vi "HFRR ADV v05 new software.vi"() -> ()   [LabVIEW 2025] (continued)
                n290 = local write "Command"(w384) -> ()
              }
              frame #2 {
                n291 = Wait (ms)(milliseconds to wait=u32 1500) -> ()  [unwired: 1 out]
              }
              frame #3 {
                n292 = local write "Command"("HE;1" ("Command")) -> ()
              }
              frame #4 {
                n293 = Wait (ms)(milliseconds to wait=u32 1500) -> ()  [unwired: 1 out]
              }
            }
          }
          frame False {
            n294 = stacked-sequence {
              frame #0 {
                n295 = Wait (ms)(milliseconds to wait=u32 1500) -> ()  [unwired: 1 out]
              }
              frame #1 {
                n296 = Concatenate Strings("ST;" ("Command"), "0" ("string")) -> (w393:string)
                n297 = local write "Command"(w393) -> ()
              }
              frame #2 {
                n298 = Wait (ms)(milliseconds to wait=u32 1500) -> ()  [unwired: 1 out]
              }
              frame #3 {
                n299 = local write "Command"("HE;0" ("Command")) -> ()
              }
              frame #4 {
                n300 = Wait (ms)(milliseconds to wait=u32 1500) -> ()  [unwired: 1 out]
              }
            }
          }
        }
      }
      event "Headen Service Button": Value Change {
        n301 = event-data() -> ()  [unwired: 1 in, 6 out]
        n302 = local read "Headen Service Button"() -> (w398:bool)
        n303 = case shown="True" w398 {
          frame False {
            n304 = property on="Password 3" class="Clust (strict)"("Visible"=FALSE) -> ()  [unwired: 2 in, 2 out]
            n305 = property on="Service Password Log" class="Str"("Visible"=FALSE) -> ()  [unwired: 2 in, 2 out]
          }
          frame True {
            n306 = property on="Password 3" class="Clust (strict)"("Visible"=TRUE) -> ()  [unwired: 2 in, 2 out]
            n307 = property on="Service Password Log" class="Str"("Visible"=TRUE) -> ()  [unwired: 2 in, 2 out]
          }
        }
      }
      event "Password 3.Service Password": Value Change {
        n308 = event-data() -> ()  [unwired: 1 in, 6 out]
        n309 = Unbundle By Name("Password 3") -> ("Service Password"=w405:string)
        n310 = call <vilib>:"Trim Whitespace.vi"("string"=w405) -> ("trimmed string"=w403:string)  [unwired: 1 in]
        n311 = Equal?(x=w403, y="Service@123") -> (x = y?=w404:bool)
        n312 = case shown="False" w404 {
          selector: w404 -> [w409 w411]
          frame False {
            n313 = local write "Service Password enable"(w409) -> ()
            n314 = property on="Service Password Log" class="Str"("Visible"=TRUE) -> ()  [unwired: 2 in, 2 out]
            n315 = property on="Tab Control 5" class="TabCtl (strict)"("Tabs Visible?"=TRUE ("Page Labels Display Visible?")) -> ()  [unwired: 2 in, 2 out]
          }
          frame True {
            n316 = property on="Service Password Log" class="Str"("Visible"=FALSE) -> ()  [unwired: 2 in, 2 out]
            "Service Password enable" <- w411
          }
        }
      }
      event "Sign In": Value Change {
        w413 = FALSE ("Visible")
        n317 = event-data() -> ()  [unwired: 1 in, 6 out]
        n318 = property on="About" class="Clust (strict)"("Visible"=w413) -> ()  [unwired: 2 in, 2 out]
        n319 = property on="Password 3" class="Clust (strict)"("Visible"=w413) -> ()  [unwired: 2 in, 2 out]
        n320 = property on="Service Password Log" class="Str"("Visible"=FALSE) -> ()  [unwired: 2 in, 2 out]
      }
      event "Info": Value Change {
        n321 = event-data() -> ()  [unwired: 1 in, 6 out]
        n322 = local read "Info"() -> (w415:bool)
        n323 = case shown="False" w415 {
          frame False {
            n324 = property on="About" class="Clust (strict)"("Visible"=FALSE) -> ()  [unwired: 2 in, 2 out]
          }
          frame True {
            n325 = property on="About" class="Clust (strict)"("Visible"=TRUE) -> ()  [unwired: 2 in, 2 out]
          }
        }
      }
      event "Calibration": Value Change {
        n326 = event-data() -> ()  [unwired: 1 in, 6 out]
        n327 = local read "Calibration"() -> (w419:bool)
        n328 = case shown="False" w419 {
          frame False {
            n329 = property on="Calibration 2" class="TabCtl (strict)"("Visible"=FALSE) -> ()  [unwired: 2 in, 2 out]
            n330 = local write "Cal Password"("" ("Cal Password")) -> ()
          }
          frame True {
            n331 = property on="Calibration 2" class="TabCtl (strict)"("Visible"=TRUE) -> ()  [unwired: 2 in, 2 out]
            n332 = local write "Cal Password"("" ("Cal Password")) -> ()
          }
        }
        n333 = property on="Wrong Password" class="Str"("Visible"=FALSE) -> ()  [unwired: 2 in, 2 out]
      }
      event "Cal Password": Value Change {
        n334 = event-data() -> ()  [unwired: 1 in, 6 out]
        n335 = local read "Cal Password"() -> (w427:string)
        n336 = call <vilib>:"Trim Whitespace.vi"("string"=w427) -> ("trimmed string"=w426:string)  [unwired: 1 in]
        n337 = Equal?(x=w426, y="Cal@321") -> (x = y?=w424:bool)
        n338 = case shown="True" w424 {
          frame False {
            n339 = property on="Wrong Password" class="Str"("Visible"=TRUE) -> ()  [unwired: 2 in, 2 out]
          }
          frame True {
            n340 = property on="Wrong Password" class="Str"("Visible"=FALSE) -> ()  [unwired: 2 in, 2 out]
            n341 = local write "Main Tab"(T2."About" ("Main Tab")) -> ()
            n342 = local write "Cal Password"("" ("Cal Password")) -> ()
            n343 = local write "Main Dashboard Buttons"(T1."About" ("Main Dashboard Buttons")) -> ()
            n344 = local write "Tab Control 5"(T7."Temperature Calibration" ("Tab Control 5")) -> ()
            n345 = property on="Calibration 2" class="TabCtl (strict)"("Visible"=FALSE) -> ()  [unwired: 2 in, 2 out]
            n346 = property on="Tab Control 5" class="TabCtl (strict)"("Tabs Visible?"=FALSE ("Page Labels Display Visible?")) -> ()  [unwired: 2 in, 2 out]
            n347 = local write "Calibration"(FALSE ("Calibration")) -> ()
          }
        }
      }
      event "Quit": Value Change {
        n348 = event-data() -> ()  [unwired: 1 in, 6 out]
      }
    }
    n349 = Wait (ms)(milliseconds to wait=u32 100) -> ()  [unwired: 1 out]
  }
  n350 = local write "Auto stop temp"(w12) -> ()
  n351 = local write "main tab sub"(enum32{"Page 1", "Page 2"}."Page 1" ("main tab sub")) -> ()
  n352 = local write "USERNAME"(w31) -> ()
  n353 = local write "Main Tab"(T2."HOME" ("Main Tab")) -> ()
  n354 = local write "USER ID"(w31) -> ()
  n355 = property on="Auto Scar Check  2" class="Clust (strict)"("Visible"=w12) -> (error out=w16:errorcluster)  [unwired: 2 in, 1 out]
  n356 = property on="Quit" class="Bool (strict)"("Value"=FALSE ("Quit")) -> (error out=w33:errorcluster)  [unwired: 2 in, 1 out]
  n357 = while {
    shift-right: [w439] -> _
    shift-left: "Enum - Selector" -> [w440]
    stop <- w441 stop-if-true
    # "Auto Start Logic Loop"
    n358 = case shown="\"close\"" w440 {
      tunnel: [w444 w450 w461 w493 w524 Auto_Start_enum."Exit" ("Enum - Selector") Auto_Start_enum."Init" ("Enum - Selector")] -> w439
      frame "Init", Default {
        n359 = local read "Auto Start Test"() -> (w443:bool)
        n360 = Select(t=Auto_Start_enum."Humidity & Temperature On" ("Enum - Selector"), s=w443, f=Auto_Start_enum."Init") -> (s? t:f=w444:T10)
      }
      frame "Humidity & Temperature On" {
        n361 = flat-sequence {
          tunnel: [Auto_Start_enum."Reach point" ("Enum - Selector")] -> w447
          frame #0 {
            w451 = T13."Disabled and Grayed Out" ("Disabled")
            w452 = TRUE ("Heater Button")
            n362 = property on="Humidity" class="Bool (strict)"("DisabledEnum"=w451) -> ()  [unwired: 2 in, 2 out]
            n363 = property on="Heater Button" class="Bool (strict)"("DisabledEnum"=w451) -> ()  [unwired: 2 in, 2 out]
            n364 = local write "Heater Button"(w452) -> ()
            n365 = local write "Humidity"(w452) -> ()
          }
          frame #1 {
            n366 = Wait (ms)(milliseconds to wait=u32 1000) -> ()  [unwired: 1 out]
          }
          frame #2 {
            w454 = TRUE ("Reach point temp")
            n367 = local write "Reach point Humidity"(w454) -> ()
            n368 = local write "Reach point temp"(w454) -> ()
          }
        }
        n369 = local read "Auto Start Test"() -> (w449:bool)
        n370 = Not(x=w449) -> (.not. x?=w448:bool)
        n371 = Select(t=Auto_Start_enum."close", s=w448, f=w447) -> (s? t:f=w450:T10)
      }
      frame "Reach point" {
        w462 = TRUE ("PAUSE")
        w470 = 1.0 ("y")
        w473 = 1.0 ("y")
        n372 = local read "Set Temperature:"() -> (w474:dbl)
        n373 = local read "Set Humidity:"() -> (w469:dbl)
        n374 = local read "Humidity ( %RH )"() -> (w475:dbl)
        n375 = Add(x=w474, y=w473) -> (x+y=w472:dbl)
        n376 = Subtract(x=w474, y=w473) -> (x-y=w471:dbl)
        n377 = Add(x=w469, y=w470) -> (x+y=w468:dbl)
        n378 = Subtract(x=w469, y=w470) -> (x-y=w467:dbl)
        n379 = local read "TEMP"() -> (w476:dbl)
        n380 = In Range and Coerce(upper limit=w468, x=w475, lower limit=w467) -> (In Range?=w456:bool)  [unwired: 1 out]
        n381 = In Range and Coerce(upper limit=w472, x=w476, lower limit=w471) -> (In Range?=w457:bool)  [unwired: 1 out]
        n382 = case shown="True" w456 {
          frame False {
          }
          frame True {
            n383 = case shown="True" "Reach point Humidity" {
              selector: "Reach point Humidity" -> [_ w482]
              frame False {
              }
              frame True {
                n384 = local read "EVENT LOG"() -> (w479:string)
                n385 = Not(x=w482) -> (.not. x?=w481:bool)
                n386 = local write "Reach point Humidity"(w481) -> ()
                n387 = call "Event Log.vi"("Content"="Target Humidity reached", "EVENT LOG"=w479) -> ("EVENT LOG"=w480:string)  [unwired: 8 in, 1 out]
                n388 = local write "EVENT LOG"(w480) -> ()
              }
            }
          }
        }
        n389 = case shown="True" w457 {
          frame False {
          }
          frame True {
            n390 = case shown="True" "Reach point temp" {
              selector: "Reach point temp" -> [_ w488]
              frame False {
              }
              frame True {
                n391 = local read "EVENT LOG"() -> (w485:string)
                n392 = Not(x=w488) -> (.not. x?=w487:bool)
                n393 = local write "Reach point temp"(w487) -> ()
                n394 = call "Event Log.vi"("Content"="Target Temperature reached", "EVENT LOG"=w485) -> ("EVENT LOG"=w486:string)  [unwired: 8 in, 1 out]
                n395 = local write "EVENT LOG"(w486) -> ()
              }
            }
          }
        }
        n396 = local read "Auto Start Test"() -> (w460:bool)
        n397 = And(x=w457, y=w456) -> (x .and. y?=w466:bool)
        n398 = Select(t=Auto_Start_enum."Maintain Stage" ("Enum - Selector"), s=w466, f=Auto_Start_enum."Reach point" ("Enum - Selector")) -> (s? t:f=w463:T10)
        n399 = Not(x=w460) -> (.not. x?=w459:bool)
        n400 = Select(t=Auto_Start_enum."close", s=w459, f=w463) -> (s? t:f=w461:T10)
        n401 = call "ELAPSED TIMER VI.vi"("RESET"=w462, "PAUSE"=w462) -> ()  [unwired: 7 in, 3 out]
      }
      frame "Maintain Stage" {
        w502 = 2.0 ("y")
        w501 = 1.0 ("y")
        # "Humidity and  temperatures Set Point  have been reached"
        n402 = local read "Set Temperature:"() -> (w508:dbl)
        n403 = local read "Set Humidity:"() -> (w505:dbl)
        n404 = local read "Humidity ( %RH )"() -> (w509:dbl)
        n405 = Add(x=w508, y=w501) -> (x+y=w507:dbl)
        n406 = Subtract(x=w508, y=w501) -> (x-y=w506:dbl)
        n407 = local read "TEMP"() -> (w510:dbl)
        n408 = Add(x=w505, y=w502) -> (x+y=w504:dbl)
        n409 = Subtract(x=w505, y=w502) -> (x-y=w503:dbl)
        n410 = In Range and Coerce(upper limit=w507, x=w510, lower limit=w506) -> (In Range?=w500:bool)  [unwired: 1 out]
        n411 = In Range and Coerce(upper limit=w504, x=w509, lower limit=w503) -> (In Range?=w499:bool)  [unwired: 1 out]
        n412 = And(x=w500, y=w499) -> (x .and. y?=w498:bool)
        n413 = Not(x=w498) -> (.not. x?=w497:bool)
        n414 = call "ELAPSED TIMER VI.vi"("TARGET"=60.0, "RESET"=w497, "PAUSE"=FALSE) -> ("ELAPSED INDICATION"=w494:bool)  [unwired: 6 in, 2 out]
        n415 = case shown="True" w494 {
          tunnel: w494 -> [_ w513]
          tunnel: [Auto_Start_enum."Maintain Stage" ("Enum - Selector") w512] -> w492
          frame False {
          }
          frame True {
            n416 = stacked-sequence {
              tunnel: w513 -> [_ _ _ _ _]
              tunnel: [_ _ _ _ Auto_Start_enum."Start Stage" ("Enum - Selector")] -> w512
              frame #0 {
                n417 = local read "EVENT LOG"() -> (w515:string)
                n418 = call "Event Log.vi"("Content"="Humidity and temperature set point has stabilized.", "EVENT LOG"=w515) -> ("EVENT LOG"=w516:string)  [unwired: 8 in, 1 out]
                n419 = local write "EVENT LOG"(w516) -> ()
              }
              frame #1 {
                n420 = Wait (ms)(milliseconds to wait=u32 100) -> ()  [unwired: 1 out]
              }
              frame #2 {
                n421 = local read "EVENT LOG"() -> (w519:string)
                n422 = call "Event Log.vi"("Content"="Auto Test Started", "EVENT LOG"=w519) -> ("EVENT LOG"=w520:string)  [unwired: 8 in, 1 out]
                n423 = local write "EVENT LOG"(w520) -> ()
              }
              frame #3 {
                w521 = TRUE ("RUN")
                n424 = local write "RUN"(w521) -> ()
                "Auto Start Temp" <- w521
              }
              frame #4 {
              }
            }
          }
        }
        n425 = local read "Auto Start Test"() -> (w491:bool)
        n426 = Not(x=w491) -> (.not. x?=w490:bool)
        n427 = Select(t=Auto_Start_enum."close", s=w490, f=w492) -> (s? t:f=w493:T10)
      }
      frame "Start Stage" {
        w523 = TRUE ("PAUSE")
        n428 = local read "Auto Start Test"() -> (w528:bool)
        n429 = Not(x=w528) -> (.not. x?=w527:bool)
        n430 = Select(t=Auto_Start_enum."close" ("Enum - Selector"), s=w527, f=Auto_Start_enum."Start Stage" ("Enum - Selector")) -> (s? t:f=w524:T10)
        n431 = call "ELAPSED TIMER VI.vi"("RESET"=w523, "PAUSE"=w523) -> ()  [unwired: 7 in, 3 out]
      }
      frame "close" {
        w529 = FALSE ("Heater Button")
        n432 = local write "RUN"(w529) -> ()
        n433 = local write "Heater Button"(w529) -> ()
        n434 = local write "Humidity"(w529) -> ()
        n435 = local write "Auto Start Test"(w529) -> ()
      }
      frame "Exit" {
      }
    }
    n436 = Wait (ms)(milliseconds to wait=u32 100) -> ()  [unwired: 1 out]
    n437 = local read "Quit"() -> (w441:bool)
  }
  n438 = property on="Service Password Log" class="Str"("Visible"=w12) -> ()  [unwired: 2 in, 2 out]
  n439 = property on="Password 3" class="Clust (strict)"("Visible"=w12) -> ()  [unwired: 2 in, 2 out]
  n440 = while {
    stop <- w558 stop-if-true
    w541 = errorcluster {"status"=FALSE, "code"=0, "source"=""} ("error in (no error) 3")
    # "this loop is for manual report generation"
    n441 = local read "Confirm Measrurement"() -> (w540:bool)
    n442 = case shown="True" w540 {
      selector: w540 -> [_ w648]
      tunnel: errorcluster {"status"=FALSE, "code"=0, "source"=""} ("error in (no error) 3") -> [_ w649]
      tunnel: [_ w647] -> _
      frame False {
      }
      frame True {
        n443 = stacked-sequence {
          tunnel: w649 -> [_ w682 _]
          tunnel: w648 -> [_ _ w789]
          tunnel: [_ w670 _] -> w647
          frame #0 {
            n444 = String To Path(string="C:\\LAB-IQ\\Image Calibrate v01.dcf") -> (path=w652:path)
            n445 = Open/Create/Replace File ("Open File")(file path (use dialog)=w652) -> (refnum out=w653:refnum<file>)  [unwired: 5 in, 2 out]
            n446 = for {
              N: 4 -> [_]
              tunnel: w653 -> [w659]
              i -> [w655]
              n447 = Read from Text File ("Read File")(file (use dialog)=w659) -> (text=w660:string)  [unwired: 3 in, 3 out]
              n448 = String Subset(string=w660, offset (0)=6, length (rest)=10 ("length (rest)")) -> (substring=w656:string)
              n449 = Fract/Exp String To Number(string=w656) -> (number=w654:dbl)  [unwired: 3 in, 1 out]
              n450 = case shown="3" w655 {
                tunnel: w654 -> [w661 w662 _ w663 _]
                frame 0 {
                  n451 = local write "5x Gain"(w661) -> ()
                }
                frame 1 {
                  n452 = local write "10x Gain"(w662) -> ()
                }
                frame 2 {
                }
                frame 3 {
                  n453 = local write "100x gain"(w663) -> ()
                }
                frame 4, Default {
                }
              }
            }
          }
          frame #1 {
            n454 = local read "TEST STANDARD"() -> (w665:T3)
            n455 = case shown="\"ISO 12156\"" w665 {
              tunnel: ["ASTM D6079" "ISO 12156"] -> w664
              frame "ASTM D6079", Default {
              }
              frame "ISO 12156" {
              }
            }
            n456 = call "IMAGE ANALYSIS.vi"("Enum"=POST_ANALYSIS_ENUM."GET MEASUREMENTS", "error in"=w682) -> ("error out"=w689:errorcluster)  [unwired: 8 in, 1 out]
            n457 = local read "Magnification :"() -> (w675:string)
            n458 = call "Stall Data Flow.vim"("value in"=w689, "milliseconds to wait"=u32 1000) -> ("value out"=w688:errorcluster)  [unwired: 1 out]
            n459 = local read "Test File List :"() -> (w686:string)
            n460 = case shown="\"10x\"" w675 {
              tunnel: [w725 w726] -> w673
              frame "5x", Default {
                n461 = local read "5x Gain"() -> (w725:dbl)
              }
              frame "10x" {
                # "5x"
                n462 = local read "10x Gain"() -> (w726:dbl)
              }
            }
            n463 = call "IMAGE ANALYSIS.vi"("Enum"=POST_ANALYSIS_ENUM."READ", "error in"=w688) -> ("error out"=w685:errorcluster, "data out"=w676:string)  [unwired: 8 in]
            n464 = Match Pattern(string=w676, regular expression="\"type\": ") -> (after substring=w680:string)  [unwired: 1 in, 3 out]
            n465 = call "IMAGE PATH CREATION PY.vi"("error in (no error)"=w685, "File Name :"=w686) -> ("error out"=w684:errorcluster, "File Path"=w672:path, "File Path String:"=w667:string)  [unwired: 7 in]
            n466 = Match Pattern(string=w680, regular expression=",") -> (before substring=w666:string)  [unwired: 1 in, 3 out]
            n467 = local read "Calibration Tab"() -> (w669:enum32{"Measrument", "Calibrate"})
            n468 = call "Stall Data Flow.vim"("value in"=w684, "milliseconds to wait"=u32 250) -> ("value out"=w668:errorcluster)  [unwired: 1 out]
            n469 = Equal?(x=w666, y="\"rectangle\"") -> (x = y?=w677:bool)
            n470 = case shown="False" w677 {
              tunnel: w676 -> [w731 w786]
              tunnel: w673 -> [_ w777]
              tunnel: cluster{"major":dbl, "minor":dbl, "average":dbl} {"major"=0.0, "minor"=0.0, "average"=0.0} -> [w729 w773]
              tunnel: [w728 w770] -> w671
              tunnel: w666 -> [w730 _]
              tunnel: w673 -> [w727 _]
              frame False {
                n471 = Equal?(x=w730, y="\"line\"") -> (x = y?=w732:bool)
                n472 = case shown="True" w732 {
                  tunnel: w731 -> [_ w747]
                  tunnel: w729 -> [w734 w746]
                  tunnel: [w734 w744] -> w728
                  tunnel: w727 -> [_ w743]
                  frame False {
                  }
                  frame True {
                    w742 = 0.0 ("Major Axis")
                    n473 = Match Pattern(string=w747, regular expression="\"length_px\":") -> (after substring=w745:string)  [unwired: 1 in, 3 out]
                    n474 = property on="Major Axis" class="DigNum (strict)"("Caption.Text"="") -> ()  [unwired: 2 in, 2 out]
                    n475 = property on="Minor Axis" class="DigNum (strict)"("Caption.Text"="") -> ()  [unwired: 2 in, 2 out]
                    n476 = property on="Average" class="DigNum (strict)"("Caption.Text"="Line") -> ()  [unwired: 2 in, 2 out]
                    n477 = Fract/Exp String To Number(string=w745, default (0 dbl)=0.0 ("default (0 DBL)")) -> (number=w741:dbl)  [unwired: 2 in, 1 out]
                    "Pixel Value" <- w741
                    n478 = Multiply(x=w741, y=w743) -> (x*y=w754:dbl)
                    n479 = Multiply(x=w754, y=1000.0) -> (x*y=w737:dbl)
                    n480 = Divide(x=w737, y=1000.0) -> (x/y=w740:dbl)
                    n481 = local write "Measurment (mm)"(w740) -> ()
                    n482 = Bundle By Name(cluster=w746, "average"=w737) -> (w744:cluster{"major":dbl, "minor":dbl, "average":dbl})
                    n483 = Number To Fractional String(number=w737, precision (6)=i16 1) -> (F-format string=w736:string)  [unwired: 2 in]
                    n484 = local write "Minor Axis"(w742) -> ()
                    n485 = local write "Major Axis"(w742) -> ()
                    n486 = Fract/Exp String To Number(string=w736) -> (number=w735:dbl)  [unwired: 3 in, 1 out]
                    n487 = local write "Average"(w735) -> ()
                  }
                }
              }
              frame True {
                w774 = 1000.0 ("y")
                w780 = 0.0 ("default (0 DBL)")
                n488 = Match Pattern(string=w786, regular expression=" \"width_px\":") -> (after substring=w784:string)  [unwired: 1 in, 3 out]
                n489 = Match Pattern(string=w784, regular expression="\"height_px\":") -> (before substring=w782:string, after substring=w781:string)  [unwired: 1 in, 2 out]
                n490 = Fract/Exp String To Number(string=w782, default (0 dbl)=w780) -> (number=w779:dbl)  [unwired: 2 in, 1 out]
                n491 = Fract/Exp String To Number(string=w781, default (0 dbl)=w780) -> (number=w778:dbl)  [unwired: 2 in, 1 out]
                n492 = Multiply(x=w779, y=w777) -> (x*y=w776:dbl)
                n493 = Multiply(x=w778, y=w777) -> (x*y=w775:dbl)
                n494 = Multiply(x=w776, y=w774) -> (x*y=w760:dbl)
                n495 = Multiply(x=w775, y=w774) -> (x*y=w758:dbl)
                n496 = Add(x=w760, y=w758) -> (x+y=w772:dbl)
                n497 = property on="Major Axis" class="DigNum (strict)"("Caption.Text"="Major Axis") -> ()  [unwired: 2 in, 2 out]
                n498 = property on="Minor Axis" class="DigNum (strict)"("Caption.Text"="Minor Axis") -> ()  [unwired: 2 in, 2 out]
                n499 = property on="Average" class="DigNum (strict)"("Caption.Text"="Average") -> ()  [unwired: 2 in, 2 out]
                n500 = Divide(x=w772, y=2.0) -> (x/y=w756:dbl)
                n501 = Bundle By Name(cluster=w773, "major"=w760, "minor"=w758, "average"=w756) -> (w770:cluster{"major":dbl, "minor":dbl, "average":dbl})
                n502 = Number To Fractional String(number=w758, precision (6)=i16 1) -> (F-format string=w765:string)  [unwired: 2 in]
                n503 = Number To Fractional String(number=w756, precision (6)=i16 1) -> (F-format string=w766:string)  [unwired: 2 in]
                n504 = Number To Fractional String(number=w760, precision (6)=i16 1) -> (F-format string=w764:string)  [unwired: 2 in]
                n505 = Fract/Exp String To Number(string=w765) -> (number=w757:dbl)  [unwired: 3 in, 1 out]
                n506 = Fract/Exp String To Number(string=w766) -> (number=w755:dbl)  [unwired: 3 in, 1 out]
                n507 = Fract/Exp String To Number(string=w764) -> (number=w759:dbl)  [unwired: 3 in, 1 out]
                n508 = local write "Major Axis"(w759) -> ()
                n509 = local write "Average"(w755) -> ()
                n510 = local write "Minor Axis"(w757) -> ()
              }
            }
            n511 = case shown="\"Measrument\", Default" w669 {
              tunnel: w672 -> [w699 _]
              tunnel: w671 -> [w698 _]
              tunnel: [w695 w724] -> w670
              tunnel: w668 -> [w697 w724]
              tunnel: w667 -> [w696 _]
              tunnel: w664 -> [w694 _]
              frame "Measrument", Default {
                n512 = stacked-sequence {
                  tunnel: w699 -> [w717 _]
                  tunnel: w698 -> [w715 _]
                  tunnel: w697 -> [w713 _]
                  tunnel: w696 -> [w712 _]
                  tunnel: [w707 _] -> w695
                  tunnel: w694 -> [w700 _]
                  frame #0 {
                    n513 = call "IMAGE ANALYSIS.vi"("Enum"=POST_ANALYSIS_ENUM."SAVE IMAGE", "error in"=w713, "IMAGE FILE PATH"=w712) -> ("error out"=w711:errorcluster)  [unwired: 7 in, 1 out]
                    n514 = call "Stall Data Flow.vim"("value in"=w711, "milliseconds to wait"=u32 1000) -> ("value out"=w702:errorcluster)  [unwired: 1 out]
                    n515 = local read "Test File List :"() -> (w719:string)
                    n516 = call "IMAGE ANALYSIS.vi"("Enum"=POST_ANALYSIS_ENUM."MINIMIZE UI", "error in"=w702) -> ("error out"=w709:errorcluster)  [unwired: 8 in, 1 out]
                    n517 = Bundle By Name(cluster=T18 {"File Name"="", "Test Method"="", "Operator"="", "Fuel Description"="", "Date and time"=""} ("Main Ref"), "Test Method"=w700, "File Name"=w719) -> (w720:T18)
                    n518 = call "Stall Data Flow.vim"("value in"=w709, "milliseconds to wait"=u32 1500) -> ("value out"=w704:errorcluster)  [unwired: 1 out]
                    n519 = call "duf file read.vi"("error in (no error)"=w704, "Main Ref"=w720) -> ("error out"=w718:errorcluster, "Main Ref 2"=w716:T18)  [unwired: 8 in]
                    n520 = call "DETECTION REPORT for manual.vi"("error in (no error)"=w718, "return value 3"=w715, "Image File Path"=w717, "Main Ref"=w716) -> ("error out"=w714:errorcluster)  [unwired: 7 in]
                    n521 = call <vilib>:"Clear Errors.vi"("error in (no error)"=w714) -> ("error out"=w705:errorcluster)  [unwired: 5 in, 1 out]
                    n522 = call "IMAGE ANALYSIS.vi"("Enum"=POST_ANALYSIS_ENUM."MINIMIZE UI", "error in"=w705) -> ("error out"=w707:errorcluster)  [unwired: 8 in, 1 out]
                  }
                  frame #1 {
                    n523 = local write "Main Tab"(T2."HOME" ("Main Tab")) -> ()
                    n524 = local write "Main Dashboard Buttons"(T1."Home" ("Main Dashboard Buttons")) -> ()
                  }
                }
              }
              frame "Calibrate" {
              }
            }
          }
          frame #2 {
            n525 = Not(x=w789) -> (.not. x?=w788:bool)
            n526 = local write "Confirm Measrurement"(w788) -> ()
            n527 = local read "Calibration Tab"() -> (w787:enum32{"Measrument", "Calibrate"})
            n528 = case shown="\"Measrument\", Default" w787 {
              frame "Measrument", Default {
                n529 = local write "Main Tab"(T2."HOME" ("Main Tab")) -> ()
              }
              frame "Calibrate" {
              }
            }
          }
        }
      }
    }
    n530 = local read "Humidity"() -> (w532:bool)
    n531 = local read "Save Change"() -> (w537:bool)
    n532 = local read "Calibrate"() -> (w538:bool)
    n533 = local read "Auto Start Test"() -> (w533:bool)
    n534 = case shown="True" w538 {
      selector: w538 -> [_ w645]
      frame False {
      }
      frame True {
        n535 = Not(x=w645) -> (.not. x?=w644:bool)
        n536 = local write "Calibrate"(w644) -> ()
        n537 = local write "Calibration Tab"(enum32{"Measrument", "Calibrate"}."Calibrate" ("Calibration Tab")) -> ()
      }
    }
    n538 = case shown="True" w537 {
      selector: w537 -> [_ w589]
      frame False {
      }
      frame True {
        n539 = stacked-sequence {
          tunnel: w589 -> [_ _ _ _ w643]
          frame #0 {
            n540 = call "IMAGE ANALYSIS.vi"("Enum"=POST_ANALYSIS_ENUM."HIDE UI") -> ()  [unwired: 9 in, 2 out]
          }
          frame #1 {
            n541 = local read "100x gain"() -> (w591:dbl)
            n542 = local read "10x Gain"() -> (w592:dbl)
            n543 = local read "5x Gain"() -> (w593:dbl)
            n544 = Number To Fractional String(number=w592, width (-)=i16 4, precision (6)=i16 7) -> (F-format string=w614:string)  [unwired: 1 in]
            n545 = Number To Fractional String(number=0.0, width (-)=i16 4, precision (6)=i16 7) -> (F-format string=w609:string)  [unwired: 1 in]
            n546 = Number To Fractional String(number=w591, width (-)=i16 4, precision (6)=i16 7) -> (F-format string=w597:string)  [unwired: 1 in]
            n547 = Number To Fractional String(number=w593, width (-)=i16 10 ("precision (6)"), precision (6)=i16 7) -> (F-format string=w623:string)  [unwired: 1 in]
            n548 = Concatenate Strings("[CH1]" ("string"), w623, " - 5x Gain" ("string"), "\r") -> (w613:string)
            n549 = Concatenate Strings("[CH2]" ("string"), w614, " - 10x Gain" ("string"), "\r") -> (w612:string)
            n550 = Concatenate Strings("[CH3]" ("string"), w609, " - 20x Gain" ("string"), "\r") -> (w603:string)
            n551 = Concatenate Strings("[CH4]" ("string"), w597, " - 100x Gain" ("string"), "\r") -> (w596:string)
            n552 = String To Path(string="C:\\LAB-IQ\\Image Calibrate v01.dcf") -> (path=w626:path)
            n553 = Concatenate Strings(w613, w612, w603, w596) -> (w611:string)
            n554 = call <vilib>:"Write Characters To File.vi"("append to file? (new file:F)"=FALSE, "character string"=w611, "file path (dialog if empty)"=w626) -> ()  [unwired: 2 in, 1 out]
          }
          frame #2 {
            n555 = String To Path(string="C:\\LAB-IQ\\Image Calibrate v01.dcf") -> (path=w629:path)
            n556 = Open/Create/Replace File ("Open File")(file path (use dialog)=w629) -> (refnum out=w630:refnum<file>)  [unwired: 5 in, 2 out]
            n557 = for {
              N: 4 -> [_]
              tunnel: w630 -> [w636]
              i -> [w632]
              n558 = Read from Text File ("Read File")(file (use dialog)=w636) -> (text=w637:string)  [unwired: 3 in, 3 out]
              n559 = String Subset(string=w637, offset (0)=6, length (rest)=10 ("length (rest)")) -> (substring=w633:string)
              n560 = Fract/Exp String To Number(string=w633) -> (number=w631:dbl)  [unwired: 3 in, 1 out]
              n561 = case shown="3" w632 {
                tunnel: w631 -> [w638 w639 _ w640 _]
                frame 0 {
                  n562 = local write "5x Gain"(w638) -> ()
                }
                frame 1 {
                  n563 = local write "10x Gain"(w639) -> ()
                }
                frame 2 {
                }
                frame 3 {
                  n564 = local write "100x gain"(w640) -> ()
                }
                frame 4, Default {
                }
              }
            }
          }
          frame #3 {
            n565 = call "IMAGE ANALYSIS.vi"("Enum"=POST_ANALYSIS_ENUM."SHOW UI") -> ()  [unwired: 9 in, 2 out]
          }
          frame #4 {
            n566 = Not(x=w643) -> (.not. x?=w642:bool)
            n567 = local write "Save Change"(w642) -> ()
          }
        }
      }
    }
    n568 = case shown="False" w533 {
      tunnel: w532 -> [w559 _]
      frame False {
        n569 = case shown="True" w559 {
          frame False {
          }
          frame True {
            n570 = local read "Set Humidity:"() -> (w563:dbl)
            n571 = local read "Set Humidity:"() -> (w566:dbl)
            n572 = local read "Humidity ( %RH )"() -> (w567:dbl)
            n573 = Subtract(x=w563, y=2.0) -> (x-y=w561:dbl)
            n574 = Add(x=w566, y=2.0) -> (x+y=w562:dbl)
            n575 = In Range and Coerce(upper limit=w562, x=w567, lower limit=w561) -> (In Range?=w560:bool)  [unwired: 1 out]
            n576 = case shown="True" w560 {
              frame False {
              }
              frame True {
                n577 = case shown="False" "Manual Humididty Reached" {
                  selector: "Manual Humididty Reached" -> [_ w570]
                  frame False {
                  }
                  frame True {
                    n578 = Not(x=w570) -> (.not. x?=w569:bool)
                    n579 = local write "Manual Humididty Reached"(w569) -> ()
                    n580 = local read "EVENT LOG"() -> (w572:string)
                    n581 = call "Event Log.vi"("Content"="Target Humidity reached", "EVENT LOG"=w572) -> ("EVENT LOG"=w571:string)  [unwired: 8 in, 1 out]
                    n582 = local write "EVENT LOG"(w571) -> ()
                  }
                }
              }
            }
          }
        }
      }
      frame True {
        n583 = local write "Manual Humididty Reached"(TRUE ("Manual Humididty Reached")) -> ()
      }
    }
    n584 = local read "Cap Live Image"() -> (w553:bool)
    n585 = local read "SCAR MEASURMENT"() -> (w556:enum32{"Auto Scar", "Manual Scar"})
    n586 = Wait (ms)(milliseconds to wait=u32 250) -> ()  [unwired: 1 out]
    n587 = Equal?(x=w556, y=enum32{"Auto Scar", "Manual Scar"}."Manual Scar" ("SCAR MEASURMENT")) -> (x = y?=w554:bool)
    n588 = And(x=w554, y=w553) -> (x .and. y?=w552:bool)
    n589 = case shown="True" w552 {
      selector: w552 -> [_ w868]
      frame False {
      }
      frame True {
        n590 = stacked-sequence {
          tunnel: [_ _ _ w883 _] -> _
          tunnel: w868 -> [_ _ _ _ w889]
          frame #0 {
            w869 = 0.0
            n591 = local write "Major Axis"(w869) -> ()
            n592 = local write "Minor Axis"(w869) -> ()
            n593 = local write "Average"(w869) -> ()
          }
          frame #1 {
            n594 = call "CAMERA LIVE FEED FGV.vi"("Enum - Menu"=CAMERA_LIVE_FEED_ENUM."CAMERA MINIMIZE") -> ()  [unwired: 9 in, 2 out]
          }
          frame #2 {
            n595 = local read "FILE 3"() -> (w877:string)
            n596 = call <vilib>:"Trim Whitespace.vi"("string"="C:\\LAB-IQ\\images\\") -> ("trimmed string"=w879:string)  [unwired: 1 in]
            n597 = String To Path(string=w879) -> (path=w878:path)
            n598 = Concatenate Strings(w877, ".png" ("string")) -> (w876:string)
            n599 = Build Path(base path=w878, name or relative path=w876) -> (appended path=w874:path)
            n600 = Path To String(path=w874) -> (string=w873:string)
            n601 = call "CAMERA LIVE FEED FGV.vi"("Enum - Menu"=CAMERA_LIVE_FEED_ENUM."CAMERA SAVE", "Image Path"=w873) -> ("error out"=w871:errorcluster)  [unwired: 8 in, 1 out]
            n602 = case shown="No Error" w871 {
              frame No Error {
                n603 = One Button Dialog(message="Image saved successfully") -> ()  [unwired: 1 in, 1 out]
              }
              frame Error {
              }
            }
          }
          frame #3 {
            n604 = call "LIST FILE NAMES.vi"() -> ("error out"=w885:errorcluster, "filenames"=w882:string[])  [unwired: 10 in]
            n605 = call "IMAGE ANALYSIS.vi"("Enum"=POST_ANALYSIS_ENUM."SHOW UI", "error in"=w885) -> ("error out"=w883:errorcluster)  [unwired: 8 in, 1 out]
            n606 = property on="Test File List :" class="CmbBox"("Strings[]"=w882) -> ()  [unwired: 2 in, 2 out]
          }
          frame #4 {
            (unwired) T19."Report" ("Main Dashboard Buttons")
            n607 = Not(x=w889) -> (.not. x?=w888:bool)
            n608 = local write "Zoom Factore"(0.0 ("Zoom Factore")) -> ()
            n609 = local write "Cap Live Image"(w888) -> ()
            n610 = local write "Main Tab"(T2."Adv Scar Report" ("Main Tab")) -> ()
            n611 = property on="Cap Live Image" class="Bool (strict)"("BoolText.Text"="Capture Image" ("Boolean Text.Text")) -> ()  [unwired: 2 in, 2 out]
            n612 = local write "Main Dashboard Buttons"(T1."Report" ("Main Dashboard Buttons")) -> ()
          }
        }
      }
    }
    n613 = local read "change Gain"() -> (w536:bool)
    n614 = local read "Back Square"() -> (w535:bool)
    n615 = case shown="True" w536 {
      selector: w536 -> [_ w580]
      frame False {
      }
      frame True {
        n616 = stacked-sequence {
          tunnel: w580 -> [_ w588]
          frame #0 {
            n617 = local read "Actual (µm)"() -> (w584:dbl)
            n618 = local read "Pixel Value"() -> (w583:dbl)
            n619 = local read "Magnification :"() -> (w582:string)
            n620 = Divide(x=w584, y=w583) -> (x/y=w581:dbl)
            n621 = case shown="\"10x\"" w582 {
              tunnel: w581 -> [w585 w586]
              frame "10x" {
                n622 = local write "10x Gain"(w585) -> ()
              }
              frame "5x", Default {
                n623 = local write "5x Gain"(w586) -> ()
              }
            }
          }
          frame #1 {
            n624 = Not(x=w588) -> (.not. x?=w587:bool)
            n625 = local write "change Gain"(w587) -> ()
          }
        }
      }
    }
    n626 = case shown="True" w535 {
      selector: w535 -> [_ w578]
      frame False {
      }
      frame True {
        n627 = Not(x=w578) -> (.not. x?=w577:bool)
        n628 = local write "Back Square"(w577) -> ()
        n629 = local write "Calibration Tab"(enum32{"Measrument", "Calibrate"}."Measrument" ("Calibration Tab")) -> ()
      }
    }
    n630 = local read "Rectangle Tool"() -> (w547:bool)
    n631 = local read "Clear ROI Tool"() -> (w546:bool)
    n632 = local read "Open Image"() -> (w551:bool)
    n633 = local read "line tool"() -> (w548:bool)
    n634 = local read "OUT"() -> (w549:bool)
    n635 = local read "In"() -> (w550:bool)
    n636 = case shown="True" w551 {
      selector: w551 -> [_ w856]
      tunnel: [w852 w858] -> _
      tunnel: w541 -> [w852 w857]
      frame False {
      }
      frame True {
        n637 = Not(x=w856) -> (.not. x?=w855:bool)
        n638 = local write "Open Image"(w855) -> ()
        n639 = call "IMAGE ANALYSIS.vi"("Enum"=POST_ANALYSIS_ENUM."HIDE UI", "error in"=w857) -> ("error out"=w865:errorcluster)  [unwired: 8 in, 1 out]
        n640 = call "File Dialog"("start path"=path "C:/LAB-IQ/images", "error in"=w865) -> ("selected path"=w854:path, "error out"=w863:errorcluster)  [unwired: 10 in, 2 out]
        "Image path  2" <- w854
        n641 = call <vilib>:"Clear Errors.vi"("error in (no error)"=w863) -> ("error out"=w862:errorcluster)  [unwired: 5 in, 1 out]
        n642 = call "IMAGE ANALYSIS.vi"("Enum"=POST_ANALYSIS_ENUM."OPEN FILE", "error in"=w862, "File Path"=w854) -> ("error out"=w861:errorcluster)  [unwired: 7 in, 1 out]
        n643 = call <vilib>:"Clear Errors.vi"("error in (no error)"=w861) -> ("error out"=w860:errorcluster)  [unwired: 5 in, 1 out]
        n644 = call "IMAGE ANALYSIS.vi"("Enum"=POST_ANALYSIS_ENUM."SHOW UI", "error in"=w860) -> ("error out"=w858:errorcluster)  [unwired: 8 in, 1 out]
        n645 = local write "Zoom Factore"(100.0 ("Zoom Factore")) -> ()
      }
    }
    n646 = case shown="True" w549 {
      selector: w549 -> [_ w837]
      tunnel: w541 -> [w834 w842]
      tunnel: [w834 w836] -> _
      frame False {
      }
      frame True {
        n647 = Not(x=w837) -> (.not. x?=w835:bool)
        n648 = local read "Zoom Factore"() -> (w840:dbl)
        n649 = local write "OUT"(w835) -> ()
        n650 = call "IMAGE ANALYSIS.vi"("Enum"=POST_ANALYSIS_ENUM."ZOOM OUT", "error in"=w842) -> ("error out"=w836:errorcluster)  [unwired: 8 in, 1 out]
        n651 = Divide(x=w840, y=1.2) -> (x/y=w838:dbl)
        n652 = local write "Zoom Factore"(w838) -> ()
      }
    }
    n653 = case shown="True" w550 {
      selector: w550 -> [_ w846]
      tunnel: w541 -> [w843 w851]
      tunnel: [w843 w844] -> _
      frame False {
      }
      frame True {
        n654 = Not(x=w846) -> (.not. x?=w845:bool)
        n655 = local read "Zoom Factore"() -> (w849:dbl)
        n656 = local write "In"(w845) -> ()
        n657 = call "IMAGE ANALYSIS.vi"("Enum"=POST_ANALYSIS_ENUM."ZOOM IN", "error in"=w851) -> ("error out"=w844:errorcluster)  [unwired: 8 in, 1 out]
        n658 = Multiply(x=w849, y=1.2) -> (x*y=w847:dbl)
        n659 = local write "Zoom Factore"(w847) -> ()
      }
    }
    n660 = case shown="True" w546 {
      selector: w546 -> [_ w818]
      tunnel: w541 -> [w816 w820]
      tunnel: [w816 w819] -> _
      frame False {
      }
      frame True {
        n661 = Not(x=w818) -> (.not. x?=w817:bool)
        n662 = local write "Clear ROI Tool"(w817) -> ()
        n663 = call "IMAGE ANALYSIS.vi"("Enum"=POST_ANALYSIS_ENUM."CLEAR ROI", "error in"=w820) -> ("error out"=w819:errorcluster)  [unwired: 8 in, 1 out]
      }
    }
    n664 = case shown="True" w548 {
      selector: w548 -> [_ w830]
      tunnel: w541 -> [w828 w833]
      tunnel: [w828 w831] -> _
      frame False {
      }
      frame True {
        n665 = Not(x=w830) -> (.not. x?=w829:bool)
        n666 = local write "line tool"(w829) -> ()
        n667 = call "IMAGE ANALYSIS.vi"("Enum"=POST_ANALYSIS_ENUM."DRAW LINE", "error in"=w833) -> ("error out"=w831:errorcluster)  [unwired: 8 in, 1 out]
      }
    }
    n668 = case shown="True" w547 {
      selector: w547 -> [_ w824]
      tunnel: w541 -> [w822 w826]
      tunnel: [w822 w825] -> _
      frame False {
      }
      frame True {
        n669 = Not(x=w824) -> (.not. x?=w823:bool)
        n670 = local write "Rectangle Tool"(w823) -> ()
        n671 = call "IMAGE ANALYSIS.vi"("Enum"=POST_ANALYSIS_ENUM."DRAW REC", "error in"=w826) -> ("error out"=w825:errorcluster)  [unwired: 8 in, 1 out]
      }
    }
    n672 = local read "SCAR MEASURMENT"() -> (w534:enum32{"Auto Scar", "Manual Scar"})
    n673 = local read "Fit to Screen Tool"() -> (w543:bool)
    n674 = local read "Resize Tool"() -> (w542:bool)
    n675 = case shown="\"Manual Scar\", Default" w534 {
      frame "Auto Scar" {
        n676 = property on="Cap Live Image" class="Bool (strict)"("BoolText.Text"="Report" ("Boolean Text.Text")) -> ()  [unwired: 2 in, 2 out]
      }
      frame "Manual Scar", Default {
        n677 = property on="Cap Live Image" class="Bool (strict)"("BoolText.Text"="Save Image" ("Boolean Text.Text")) -> ()  [unwired: 2 in, 2 out]
      }
    }
    n678 = local read "ROI Color Tool"() -> (w544:bool)
    n679 = local read "Pan Tool"() -> (w545:bool)
    n680 = case shown="True" w545 {
      selector: w545 -> [_ w812]
      tunnel: w541 -> [w810 w814]
      tunnel: [w810 w813] -> _
      frame False {
      }
      frame True {
        n681 = Not(x=w812) -> (.not. x?=w811:bool)
        n682 = call "IMAGE ANALYSIS.vi"("Enum"=POST_ANALYSIS_ENUM."PAN", "error in"=w814) -> ("error out"=w813:errorcluster)  [unwired: 8 in, 1 out]
        n683 = local write "Pan Tool"(w811) -> ()
      }
    }
    n684 = case shown="True" w542 {
      selector: w542 -> [_ w796]
      tunnel: w541 -> [w791 w793]
      tunnel: [w791 w792] -> _
      frame False {
      }
      frame True {
        n685 = Not(x=w796) -> (.not. x?=w795:bool)
        n686 = local write "Resize Tool"(w795) -> ()
        n687 = call "IMAGE ANALYSIS.vi"("Enum"=POST_ANALYSIS_ENUM."RESIZE MODE", "error in"=w793) -> ("error out"=w792:errorcluster)  [unwired: 8 in, 1 out]
      }
    }
    n688 = case shown="True" w543 {
      selector: w543 -> [_ w801]
      tunnel: [w797 w802] -> _
      tunnel: w541 -> [w797 w800]
      frame False {
      }
      frame True {
        n689 = Not(x=w801) -> (.not. x?=w799:bool)
        n690 = local write "Zoom Factore"(100.0 ("Zoom Factore")) -> ()
        n691 = local write "Fit to Screen Tool"(w799) -> ()
        n692 = call "IMAGE ANALYSIS.vi"("Enum"=POST_ANALYSIS_ENUM."FIT", "error in"=w800) -> ("error out"=w802:errorcluster)  [unwired: 8 in, 1 out]
      }
    }
    n693 = case shown="True" w544 {
      selector: w544 -> [_ w807]
      tunnel: [w804 w808] -> _
      tunnel: w541 -> [w804 w805]
      frame False {
      }
      frame True {
        n694 = Not(x=w807) -> (.not. x?=w806:bool)
        n695 = local write "ROI Color Tool"(w806) -> ()
        n696 = call "IMAGE ANALYSIS.vi"("Enum"=POST_ANALYSIS_ENUM."SET ROI COLOR", "error in"=w805) -> ("error out"=w808:errorcluster)  [unwired: 8 in, 1 out]
      }
    }
    n697 = local read "Quit"() -> (w558:bool)
  }
  n698 = while {
    stop <- w892 stop-if-true
    n699 = local read "Image Path"() -> (w895:path)
    n700 = local read "Print 3"() -> (w898:bool)
    n701 = Equal?(x=w895, y=path "") -> (x = y?=w894:bool)
    n702 = Not(x=w894) -> (.not. x?=w893:bool)
    n703 = property on="Print 3" class="Bool (strict)"("Visible"=w893) -> ()  [unwired: 2 in, 2 out]
    n704 = case shown="True" w898 {
      frame False {
        n705 = local write "Rd"(TRUE ("Boolean 7")) -> ()
      }
      frame True {
        n706 = flat-sequence {
          tunnel: [w938] -> w906
          tunnel: [w925] -> w904
          tunnel: [w935] -> w900
          tunnel: w906 -> [w947]
          tunnel: [w947] -> w905
          tunnel: w904 -> [w946]
          tunnel: [w946] -> w903
          tunnel: [w944] -> w902
          tunnel: [w943] -> w901
          tunnel: w900 -> [w943]
          tunnel: w905 -> [w949]
          tunnel: w903 -> [w950]
          tunnel: w902 -> [_]
          tunnel: w901 -> [w948]
          frame #0 {
            n707 = case shown="True" "Rd" {
              frame False {
              }
              frame True {
                n708 = while {
                  tunnel: "abcdefABCDEF" ("string 2") -> [w917]
                  shift-right: [w915] -> w909
                  shift-left: "" -> [w914]
                  i -> [w924]
                  stop <- w923 stop-if-true
                  n709 = Random Number (0-1)() -> (number: 0 to 1=w918:dbl)
                  n710 = Multiply(x=w918, y=62.0) -> (x*y=w920:dbl)
                  n711 = Decrement(x="Length 2") -> (x-1=w913:i16)
                  n712 = To Word Integer(number=w920) -> (16bit integer=w921:i16)
                  n713 = String Subset(string=w917, offset (0)=w921, length (rest)=1 ("length (rest)")) -> (substring=w916:string)
                  n714 = Greater Or Equal?(x=w924, y=w913) -> (x >= y?=w923:bool)
                  n715 = Concatenate Strings(w916, w914) -> (w915:string)
                }
                "String 10" <- w909
                n716 = local write "Rd"(FALSE ("Boolean 7")) -> ()
              }
            }
          }
          frame #1 {
            w936 = "_resized.jpg" ("command line")
            (unwired) ".jpg -resize 320x240 " ("string")
            (unwired) "Choose an Image File" ("prompt")
            # "-resize 1798x425"
            n717 = local read "Image Path"() -> (w930:path)
            n718 = Strip Path(path=w930) -> (stripped path=w925:path, name=w926:string)
            n719 = Match Pattern(string=w926, regular expression=".jpg") -> (before substring=→"before substring 2":string, after substring=→"after substring":string)  [unwired: 1 in, 2 out]
            n720 = Match Pattern(string=w926, regular expression="\\") -> (before substring=w932:string)  [unwired: 1 in, 3 out]
            n721 = Match Pattern(string=w932, regular expression=".jpg") -> (before substring=w931:string)  [unwired: 1 in, 3 out]
            n722 = Concatenate Strings("cmd /c convert " ("string"), w931, ".jpg -resize 320x240  " ("command line"), w931, w936) -> (w939:string)
            n723 = call <vilib>:"System Exec.vi"("run minimized? (F)"=TRUE, "wait until completion? (T)"=TRUE, "working directory"=w925, "command line"=w939) -> ("error out"=w938:errorcluster)  [unwired: 4 in, 3 out]
            "error out 2" <- w938
            n724 = Concatenate Strings(w931, w936) -> (w935:string)
          }
          frame #2 {
            n725 = Wait (ms)(milliseconds to wait=u32 2000 ("millisecond timer value")) -> (millisecond timer value=w944:u32)
          }
          frame #3 {
            n726 = case shown="No Error" w949 {
              tunnel: w950 -> [w953 _]
              tunnel: w948 -> [w951 _]
              frame No Error {
                (unwired) ".jpg" ("string")
                n727 = Path To String(path=w953) -> (string=w957:string)
                n728 = Concatenate Strings(w957, "\\" ("string"), w951) -> (w956:string)
                n729 = String To Path(string=w956) -> (path=w955:path)
                n730 = call <vilib>:"Read JPEG File.vi"("path to JPEG file"=w955) -> ("image data"=w959:T11)  [unwired: 8 in, 2 out]
                "image data" <- w959
                n731 = local write "Print 3"(FALSE ("Print 2")) -> ()
                n732 = call <vilib>:"Draw Flattened Pixmap.vi"("image data"=w959) -> ("new picture"=→"new picture":picture)  [unwired: 8 in]
              }
              frame Error {
              }
            }
          }
        }
      }
    }
    n733 = Wait (ms)(milliseconds to wait=u32 20 ("millisecond timer value")) -> ()  [unwired: 1 out]
    n734 = local read "Quit"() -> (w892:bool)
  }
  n735 = while {
    tunnel: w33 -> [_]
    tunnel: w16 -> [_]
    stop <- w990 stop-if-true
    # "New Adv Logics"
    n736 = local read "Main Tab"() -> (w969:T2)
    n737 = local read "Main Tab"() -> (w988:T2)
    n738 = local read "Sign In"() -> (w987:bool)
    n739 = case shown="\"Adv Scar\"" w969 {
      frame "HOME", Default {
        n740 = local read "LIVE FEED MIN TEMP"() -> (w1117:bool)
        n741 = local write "LIVE FEED MAX TEMP"(TRUE ("LIVE FEED MAX TEMP")) -> ()
        n742 = local read "CAMERA ROI MIN TEMP"() -> (w1115:bool)
        n743 = case shown="True" w1117 {
          selector: w1117 -> [_ w1124]
          frame False {
          }
          frame True {
            n744 = Not(x=w1124) -> (.not. x?=w1123:bool)
            n745 = local write "LIVE FEED MIN TEMP"(w1123) -> ()
            n746 = call "CAMERA LIVE FEED FGV.vi"("Enum - Menu"=CAMERA_LIVE_FEED_ENUM."CAMERA MINIMIZE") -> ()  [unwired: 9 in, 2 out]
          }
        }
        n747 = case shown="True" w1115 {
          selector: w1115 -> [_ w1121]
          frame False {
          }
          frame True {
            n748 = Not(x=w1121) -> (.not. x?=w1120:bool)
            n749 = local write "CAMERA ROI MIN TEMP"(w1120) -> ()
            n750 = call "IMAGE ANALYSIS.vi"("Enum"=POST_ANALYSIS_ENUM."MINIMIZE UI") -> ()  [unwired: 9 in, 2 out]
          }
        }
        n751 = local write "CAMERA ROI MAX TEMP"(TRUE ("CAMERA ROI MAX TEMP")) -> ()
      }
      frame "Test Setup" {
        n752 = local read "LIVE FEED MIN TEMP"() -> (w1127:bool)
        n753 = local read "CAMERA ROI MIN TEMP"() -> (w1125:bool)
        n754 = local write "LIVE FEED MAX TEMP"(TRUE ("LIVE FEED MAX TEMP")) -> ()
        n755 = case shown="True" w1127 {
          selector: w1127 -> [_ w1134]
          frame False {
          }
          frame True {
            n756 = Not(x=w1134) -> (.not. x?=w1133:bool)
            n757 = local write "LIVE FEED MIN TEMP"(w1133) -> ()
            n758 = call "CAMERA LIVE FEED FGV.vi"("Enum - Menu"=CAMERA_LIVE_FEED_ENUM."CAMERA MINIMIZE") -> ()  [unwired: 9 in, 2 out]
          }
        }
        n759 = case shown="True" w1125 {
          selector: w1125 -> [_ w1131]
          frame False {
          }
          frame True {
            n760 = Not(x=w1131) -> (.not. x?=w1130:bool)
            n761 = local write "CAMERA ROI MIN TEMP"(w1130) -> ()
            n762 = call "IMAGE ANALYSIS.vi"("Enum"=POST_ANALYSIS_ENUM."MINIMIZE UI") -> ()  [unwired: 9 in, 2 out]
          }
        }
        n763 = local write "CAMERA ROI MAX TEMP"(TRUE ("CAMERA ROI MAX TEMP")) -> ()
      }
      frame "Acquire" {
        n764 = local read "LIVE FEED MIN TEMP"() -> (w1137:bool)
        n765 = local write "LIVE FEED MAX TEMP"(TRUE ("LIVE FEED MAX TEMP")) -> ()
        n766 = local read "CAMERA ROI MIN TEMP"() -> (w1135:bool)
        n767 = case shown="True" w1137 {
          selector: w1137 -> [_ w1144]
          frame False {
          }
          frame True {
            n768 = Not(x=w1144) -> (.not. x?=w1143:bool)
            n769 = local write "LIVE FEED MIN TEMP"(w1143) -> ()
            n770 = call "CAMERA LIVE FEED FGV.vi"("Enum - Menu"=CAMERA_LIVE_FEED_ENUM."CAMERA MINIMIZE") -> ()  [unwired: 9 in, 2 out]
          }
        }
        n771 = case shown="True" w1135 {
          selector: w1135 -> [_ w1141]
          frame False {
          }
          frame True {
            n772 = Not(x=w1141) -> (.not. x?=w1140:bool)
            n773 = local write "CAMERA ROI MIN TEMP"(w1140) -> ()
            n774 = call "IMAGE ANALYSIS.vi"("Enum"=POST_ANALYSIS_ENUM."MINIMIZE UI") -> ()  [unwired: 9 in, 2 out]
          }
        }
        n775 = local write "CAMERA ROI MAX TEMP"(TRUE ("CAMERA ROI MAX TEMP")) -> ()
      }
      frame "Adv Scar" {
        n776 = local read "CAMERA ROI MIN TEMP"() -> (w1145:bool)
        n777 = case shown="True" "LIVE FEED MAX TEMP" {
          selector: "LIVE FEED MAX TEMP" -> [_ w1166]
          frame False {
          }
          frame True {
            n778 = Not(x=w1166) -> (.not. x?=w1165:bool)
            n779 = local write "LIVE FEED MAX TEMP"(w1165) -> ()
            n780 = call "CAMERA LIVE FEED FGV.vi"("Enum - Menu"=CAMERA_LIVE_FEED_ENUM."CAMERA RESTORE") -> ("error out"=w1156:errorcluster)  [unwired: 9 in, 1 out]
            n781 = Type Cast(type=30, x=0) -> (*(type *) &x=w1160:i32)
            n782 = Add(x=w1160, y=48) -> (x+y=w1161:i32)
            n783 = call "CAMERA LIVE FEED FGV.vi"("Enum - Menu"=CAMERA_LIVE_FEED_ENUM."CAMERA MODE SET", "error in (no error)"=w1156, "CAMERA MODE"=w1161) -> ("error out"=w1153:errorcluster)  [unwired: 7 in, 1 out]
            n784 = call "CAMERA LIVE FEED FGV.vi"("Enum - Menu"=CAMERA_LIVE_FEED_ENUM."CAMERA GRAY", "error in (no error)"=w1153) -> ("error out"=w1152:errorcluster)  [unwired: 8 in, 1 out]
            n785 = call "LIST FILE NAMES.vi"("error in (no error)"=w1152) -> ("error out"=w1162:errorcluster, "filenames"=w1163:string[])  [unwired: 9 in]
            n786 = property on="FILE 3" class="CmbBox"(error in=w1162, "Strings[]"=w1163) -> ()  [unwired: 1 in, 2 out]
          }
        }
        n787 = case shown="True" w1145 {
          selector: w1145 -> [_ w1151]
          frame False {
          }
          frame True {
            n788 = Not(x=w1151) -> (.not. x?=w1150:bool)
            n789 = local write "CAMERA ROI MIN TEMP"(w1150) -> ()
            n790 = call "IMAGE ANALYSIS.vi"("Enum"=POST_ANALYSIS_ENUM."MINIMIZE UI") -> ()  [unwired: 9 in, 2 out]
          }
        }
        n791 = local write "CAMERA ROI MAX TEMP"(TRUE ("CAMERA ROI MAX TEMP")) -> ()
        "LIVE FEED MIN TEMP" <- TRUE ("LIVE FEED MIN TEMP")
      }
      frame "Adv Scar Report" {
        n792 = local read "CAMERA ROI MAX TEMP"() -> (w1167:bool)
        n793 = local read "LIVE FEED MIN TEMP"() -> (w1169:bool)
        n794 = local write "LIVE FEED MAX TEMP"(TRUE ("LIVE FEED MAX TEMP")) -> ()
        n795 = case shown="True" w1169 {
          selector: w1169 -> [_ w1178]
          frame False {
          }
          frame True {
            n796 = Not(x=w1178) -> (.not. x?=w1177:bool)
            n797 = local write "LIVE FEED MIN TEMP"(w1177) -> ()
            n798 = call "CAMERA LIVE FEED FGV.vi"("Enum - Menu"=CAMERA_LIVE_FEED_ENUM."CAMERA MINIMIZE") -> ()  [unwired: 9 in, 2 out]
          }
        }
        n799 = case shown="True" w1167 {
          selector: w1167 -> [_ w1175]
          frame False {
          }
          frame True {
            n800 = Not(x=w1175) -> (.not. x?=w1173:bool)
            n801 = local write "CAMERA ROI MAX TEMP"(w1173) -> ()
            n802 = call "IMAGE ANALYSIS.vi"("Enum"=POST_ANALYSIS_ENUM."SHOW UI") -> ("error out"=w1172:errorcluster)  [unwired: 9 in, 1 out]
            n803 = call "LIST FILE NAMES.vi"("error in (no error)"=w1172) -> ("filenames"=w1171:string[])  [unwired: 9 in, 1 out]
            n804 = property on="Test File List :" class="CmbBox"("Strings[]"=w1171) -> ()  [unwired: 2 in, 2 out]
          }
        }
        n805 = local write "CAMERA ROI MIN TEMP"(TRUE ("CAMERA ROI MIN TEMP")) -> ()
      }
      frame "Compare Files" {
